vi "3DS Model to Vertex Array.vi"(10 "FaceList":cluster{"v1":i32, "v2":i32, "v3":i32}[](array[cluster]), 11 "Array":T1[](array[typedef]) {"z" format="%.2f"; "y" format="%.2f"; "x" format="%.2f"}) -> (1 "point3f 2":sgl[](array[numeric]), 2 "point3f 3":sgl[](array[numeric]), 3 "point3f":sgl[](array[numeric]), 4 "Count":i32)   [LabVIEW 2026, in "3D utilities.lvlib"]
uses:
  3D utilities.lvlib
  <vilib>/picture/3D Picture Control/Old 3D Toolkit.llb/point3f.ctl
  <vilib>/picture/3D Picture Control/NI_Old 3D Toolkit.lvlib
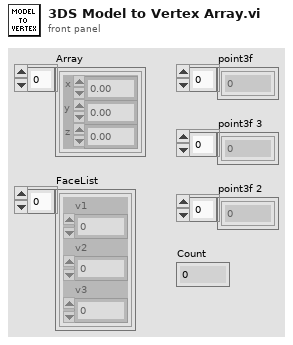
[diagram p1: front panel]
types:
  T1 = typedef "NI_3D Picture Control.lvlib/NI_Old 3D Toolkit.lvlib/point3f.ctl" = cluster{"x":sgl, "y":sgl, "z":sgl}
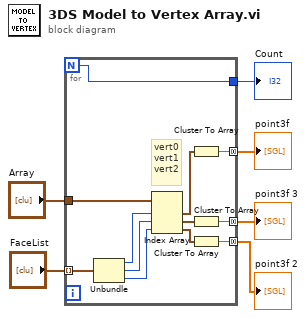
[diagram p0: block diagram]
diagram:
  n1 = for {
    N -> [w7]
    tunnel: "Array" -> [w12]
    tunnel: "FaceList" -> [w11] mode=indexing
    tunnel: [w10] -> w5 mode=concatenating
    tunnel: [w9] -> w3 mode=concatenating
    tunnel: [w8] -> w4 mode=concatenating
    tunnel: [w7] -> w6
    # "vert0\nvert1\nvert2"
    n2 = Unbundle(w11) -> ("v1"=w13:i32, "v2"=w14:i32, "v3"=w15:i32)
    n3 = Index Array(array=w12, index #1=w13, index #2=w14, index #3=w15) -> (element #1=w16:T1, element #2=w17:T1, element #3=w18:T1)
    n4 = Cluster To Array(cluster=w16) -> (array=w10:sgl[])
    n5 = Cluster To Array(cluster=w17) -> (array=w9:sgl[])
    n6 = Cluster To Array(cluster=w18) -> (array=w8:sgl[])
  }
  "Count" <- w6
  "point3f" <- w5
  "point3f 2" <- w4
  "point3f 3" <- w3
